vi "Shutdown.vi"(8 "error in":errorcluster, 11 "cCRDS_new in":refnum<class "cCRDS.lvclass">=refnum) -> (0 "error out":errorcluster, 3 "cCRDS_new out":refnum<class "cCRDS.lvclass">)   [LabVIEW 2015, in "cCRDS.lvclass"]
uses:
  cCRDS.lvclass
  cCRDS.lvclass/cCRDS.ctl
  Reusable/CRDS/Main/CRDS.lvclass
  <resource>/objmgr/daqmx.rc
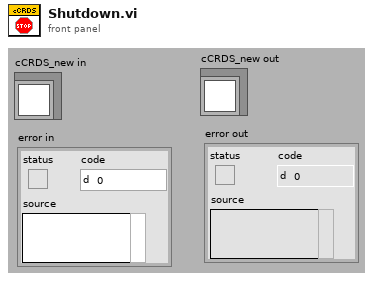
[diagram p1: front panel]
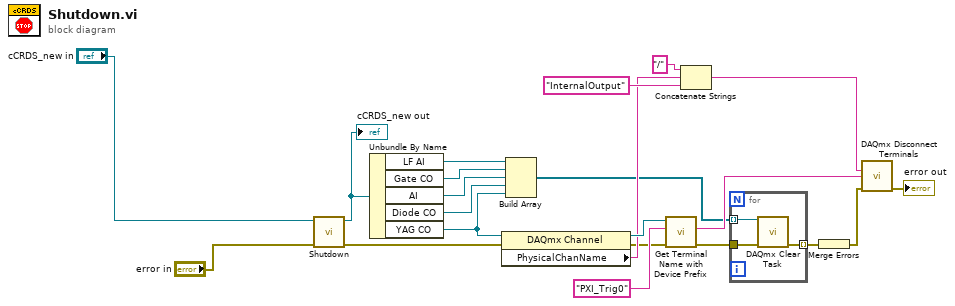
[diagram p0: block diagram]
diagram:
  n1 = call-parent "Shutdown.vi"("error in"="error in", "Instrument in"="cCRDS_new in") -> ("error out"=w5:errorcluster, "Instrument out"=w3:refnum<class "cCRDS.lvclass">)  [unwired: 8 in]
  "cCRDS_new out" <- w3
  n2 = Unbundle By Name(w3) -> ("LF AI"=w11:refnum<k21>, "Gate CO"=w10:refnum<k21>, "AI"=w9:refnum<k21>, "Diode CO"=w8:refnum<k21>, "YAG CO"=w7:refnum<k21>)
  n3 = property class="DAQmx Channel"(reference=w7, error in=w5) -> (reference out=w15:refnum<k21>, error out=w13:errorcluster, "PhysicalChanName"=w14:tag)
  n4 = Build Array(w11, w10, w9, w8, w7) -> (w6:refnum<k21>[])
  n5 = call "Get Terminal Name with Device Prefix.vi"("error in"=w13, "Local Terminal Name"="PXI_Trig0", "task/channels in"=w15) -> ("error out"=w12:errorcluster, "Terminal Name with Device Prefix"=w22:tag)  [unwired: 6 in, 1 out]
  n6 = Concatenate Strings("/", w14, "InternalOutput" ("string")) -> (w21:string)
  n7 = for {
    tunnel: w6 -> [w23] mode=indexing
    tunnel: [w25] -> w16 mode=indexing
    tunnel: w12 -> [w24]
    n8 = call <vilib>:"DAQmx Clear Task.vi"("task in"=w23, "error in"=w24) -> ("error out"=w25:errorcluster)  [unwired: 13 in]
  }
  n9 = Merge Errors(w16) -> (w20:errorcluster)
  n10 = call <vilib>:"DAQmx Disconnect Terminals.vi"("source terminal"=w21, "destination terminal"=w22, "error in"=w20) -> ("error out"=→"error out":errorcluster)  [unwired: 12 in]
